vi "XML Script - GrowableNode.vi"   [LabVIEW 2020]
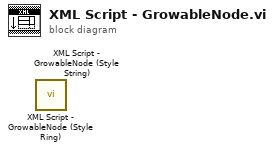
[diagram p0: block diagram]
diagram:
  n1 = call <vilib>:"XML Script - GrowableNode (Style Ring).vi"() -> ()  [unwired: 10 in, 2 out]
  n2 = call <vilib>:"XML Script - GrowableNode (Style String).vi"() -> ()  [unwired: 10 in, 2 out]
